vi "Get Initial Source Voltage.vi"(1 "measurement configuration":T1={"Mode of operation"=enum."Perform measurement", "DUT setup time"=1.0, "Source delay"=0.005, "Aperture time"=0.005, "Nominal output voltage"=3.3, "Source pin name"="", "Source sense"=1009, "Source current limit"=25.0, "Source maximum power"=300.0, "Source start voltage"=5.0, "Source stop voltage"=20.0, "Source voltage sweep points"=10, "Use Source voltage array"=FALSE, "Source voltage array"=[], "Load pin name"="", "Load sense"=1009, "Load voltage limit range"=6.0, "Load sweep type"="Logarithmic", "Load start current"=0.1, "Load stop current"=24.0, "Load current sweep points/points per decade"=10, "Use Load current array"=FALSE, "Load current array"=[], "Pin Names for Scope"=[], "vertical range"=[], "vertical offset"=[], "probe attenuation"=[], "vertical coupling"=[], "channel enabled"=[], "input impedance"=[], "max input frequency"=[], "min sample rate"=[], "reference position"=[], "min record length"=[], "enforce realtime"=[]} {"input impedance" items=["1 mega ohm"=0, "50 ohms"=2]; "vertical coupling" items=["AC", "DC", "Ground"]; "Load sense" items=["Local"=1008, "Remote"=1009]; "Source sense" items=["Local"=1008, "Remote"=1009]}) -> (0 "Initial Source Voltage":dbl)   [LabVIEW 2021, in "Efficiency And Load Regulation with Pin Map.lvlib"]
uses:
  Efficiency And Load Regulation with Pin Map.lvlib
  <instrlib>/niScope/Controls/niScope vertical coupling.ctl
  Measurement Configuration.ctl
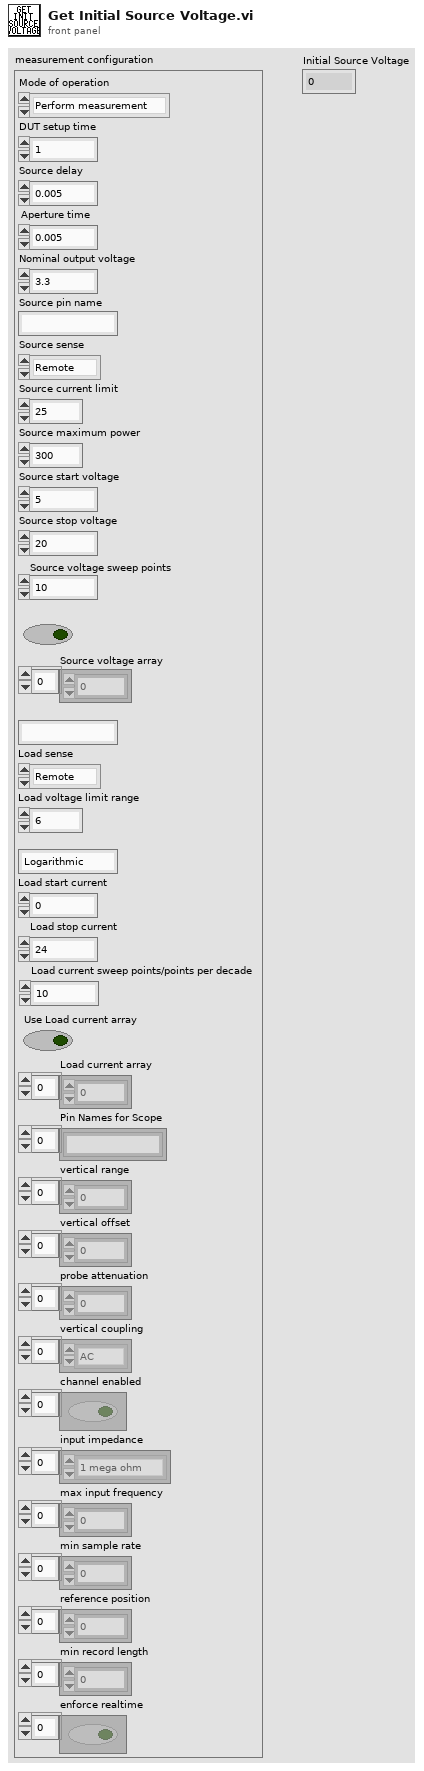
[diagram p1: front panel]
types:
  T1 = typedef "Efficiency And Load Regulation with Pin Map.lvlib/Measurement Configuration.ctl" = cluster{"Mode of operation":enum32{"Power on the DUT", "Perform measurement", "Power off the DUT"}, "DUT setup time":dbl, "Source delay":dbl, "Aperture time":dbl, "Nominal output voltage":dbl, "Source pin name":string, "Source sense":i32, "Source current limit":dbl, "Source maximum power":dbl, "Source start voltage":dbl, "Source stop voltage":dbl, "Source voltage sweep points":i32, "Use Source voltage array":bool, "Source voltage array":dbl[], "Load pin name":string, "Load sense":i32, "Load voltage limit range":dbl, "Load sweep type":string, "Load start current":dbl, "Load stop current":dbl, "Load current sweep points/points per decade":i32, "Use Load current array":bool, "Load current array":dbl[], "Pin Names for Scope":string[], "vertical range":dbl[], "vertical offset":dbl[], "probe attenuation":dbl[], "vertical coupling":T2[], "channel enabled":bool[], "input impedance":u32[], "max input frequency":dbl[], "min sample rate":dbl[], "reference position":dbl[], "min record length":i32[], "enforce realtime":bool[]}
  T2 = typedef "niScope vertical coupling.ctl" = i32
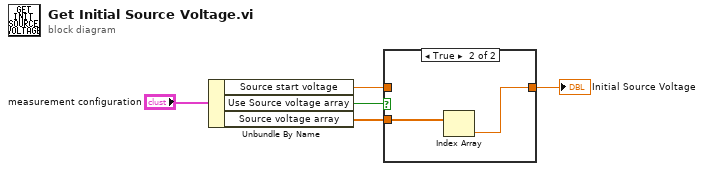
[diagram p0: block diagram]
diagram:
  n1 = Unbundle By Name("measurement configuration") -> ("Source start voltage"=w3:dbl, "Use Source voltage array"=w4:bool, "Source voltage array"=w2:dbl[])
  n2 = case shown="True" w4 {
    tunnel: w3 -> [w6 _]
    tunnel: w2 -> [_ w8]
    tunnel: [w6 w7] -> w1
    frame False {
    }
    frame True {
      n3 = Index Array(array=w8) -> (element=w7:dbl)  [unwired: 1 in]
    }
  }
  "Initial Source Voltage" <- w1
